vi "ep_Lead or Lag.vi"(8 "error in (no error)":errorcluster, 10 "current fundamental vectors":cdb[](array[numeric]), 11 "voltage fundamental vectors":cdb[](array[numeric])) -> (0 "error out":errorcluster, 3 "lead/lag ? (T)":bool[](array[boolean]))   [LabVIEW 2024]
doc: "Detects if the voltage signal is leading or lagging the current signal."
uses:
  <vilib>/Analysis/coordinate.llb/Angle Units.ctl
  <vilib>/Analysis/coordinate.llb/Wrap Angle (array).vi
  <vilib>/Analysis/NI_AAL_Angle.lvlib
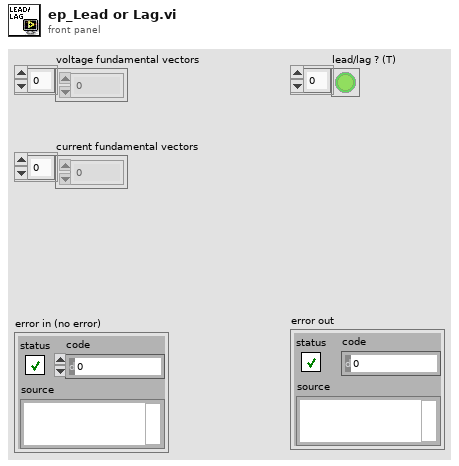
[diagram p1: front panel]
types:
  T1 = typedef "NI_AAL_Angle.lvlib/Angle Units.ctl" = i32
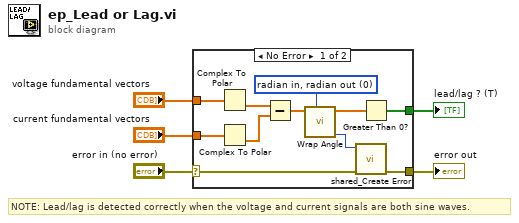
[diagram p0: block diagram]
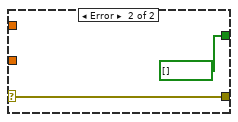
[diagram p2: hidden frame]
diagram:
  # "NOTE: Lead/lag is detected correctly when the voltage and current signals are both sine waves."
  n1 = case shown="No Error" "error in (no error)" {
    selector: "error in (no error)" -> [w11 w18]
    tunnel: "current fundamental vectors" -> [w16 _]
    tunnel: "voltage fundamental vectors" -> [w15 _]
    tunnel: [w8 w18] -> w4
    tunnel: [w6 bool[] []] -> w1
    frame No Error {
      w9 = T1 0 items=["radian in, radian out", "radian in, degree out", "degree in, degree out", "degree in, radian out"] ("angle units")
      n2 = Complex To Polar(r * e^(i*theta)=w15) -> (theta=w14:dbl[])  [unwired: 1 out]
      n3 = Complex To Polar(r * e^(i*theta)=w16) -> (theta=w13:dbl[])  [unwired: 1 out]
      n4 = Subtract(x=w14, y=w13) -> (x-y=w12:dbl[])
      n5 = call-poly <vilib>:"Wrap Angle.vi"("angle units"=w9, "Angle In"=w12) -> ("error"=w10:i32, "Angle Out"=w7:dbl[])  [unwired: 8 in]
      n6 = call <vilib>:"shared_Create Error.vi"("error in (no error)"=w11, "error code (0)"=w10) -> ("error out"=w8:errorcluster)  [unwired: 9 in]
      n7 = Greater Than 0?(x=w7) -> (x > 0?=w6:bool[])
    }
    frame Error {
    }
  }
  "error out" <- w4
  "lead/lag ? (T)" <- w1
